vi "Encoder Rate.vi"() -> ()   [LabVIEW 2016]
panel:
  in  "Numeric":dbl
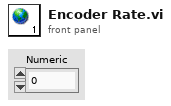
[diagram p1: front panel]
diagram:
